vi "setSweepConfiguration.vi"(8 "error in (no error)":errorcluster, 10 "setSweepConfiguration":variant, 11 "Instrument.LockinAPI in":refnum<class "Instrument.LockinAPI.lvclass">) -> (0 "error out":errorcluster, 3 "Instrument.LockinAPI out":refnum<class "Instrument.LockinAPI.lvclass">)   [LabVIEW 2019, in "Instrument.LockinAPI.lvclass"]
doc: "Configure Sweep mode"
uses:
  Instrument.LockinAPI.lvclass
  C:/Users/patrick/Documents/GitHub/Instrument-Framework/lvsrc/Instrument/Instrument.lvclass
  Typedefs/API/LockinAPI.Commands--Enum.ctl
  de6fb303-8df8-49ef-b17e-c3f9f1bf9765.vi
  de6fb303-8df8-49ef-b17e-c3f9f1bf9765.vi/18aa9fab-8d34-42d7-9854-65ef5eaa2568.vi
  de6fb303-8df8-49ef-b17e-c3f9f1bf9765.vi/18aa9fab-8d34-42d7-9854-65ef5eaa2568.vi/384e9f5b-745a-4fe9-8395-b24d125153c2.vi
  de6fb303-8df8-49ef-b17e-c3f9f1bf9765.vi/18aa9fab-8d34-42d7-9854-65ef5eaa2568.vi/384e9f5b-745a-4fe9-8395-b24d125153c2.vi/a2febbde-3d5a-455a-bb03-93f8f6d728bf.vi
  de6fb303-8df8-49ef-b17e-c3f9f1bf9765.vi/18aa9fab-8d34-42d7-9854-65ef5eaa2568.vi/384e9f5b-745a-4fe9-8395-b24d125153c2.vi/28684123-1cf5-4cee-a4b2-57f2f2fe93a2.vi
  Instrument/Protected/Validate API method.vi
  Instrument/Private/Get RC Connection Status.vi
  Instrument/API/Send and Receive.vi
  <vilib>/Utility/Data Type/Get Type Information.vi
  <vilib>/JDP Science/JSONtext/JSON text to Variant.vi
  <vilib>/JDP Science/JSONtext/LVClass Serializer/JSONtext LVClass Serializer.lvclass
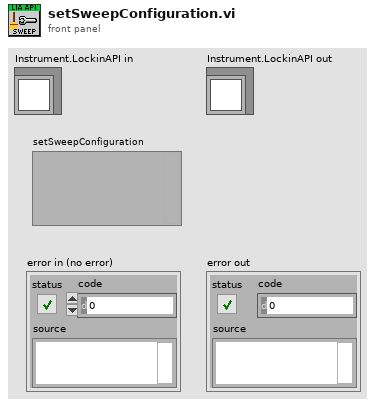
[diagram p1: front panel]
types:
  T1 = typedef "Instrument.LockinAPI.lvclass/LockinAPI.Commands--Enum.ctl" = enum16{"setAI", "setAO", "setAO_Amplitude", "setAO_DC", "setAO_Frequency", "setAO_Phase", "setAO_Function", "setAO_I+", "setREF", "setREF_Frequency", "setREF_Phase", "setREF_TC", "setREF_Roll-Off", "setDAQ", "setSampling", "setOffset", "setState", "getState", "getAO", "getAI", "getResults", "getSampling", "getAOconfig", "getREFconfig", "setInputGain", "setOutputGain", "getInputGain", "getOutputGain", "setSamplingMode", "getSamplingMode", "setSweep", "setSweepTime", "setSweepTable", "getStatus", "getSweepResults", "getSweepWaveforms", "startSweep", "stopSweep", "setAUX", "getAUX"}
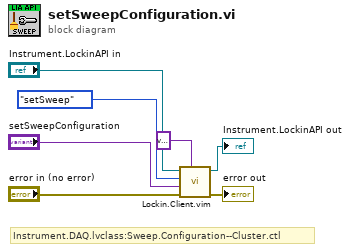
[diagram p0: block diagram]
diagram:
  # "Instrument.DAQ.lvclass:Sweep.Configuration--Cluster.ctl"
  n1 = call "Lockin.Client.vim"("Data Out type"=variant, "error in (no error)"="error in (no error)", "Data"="setSweepConfiguration", "Command"=LockinAPI.Commands--Enum."setSweep", "Instrument.LockinAPI in"="Instrument.LockinAPI in") -> ("error out"=→"error out":errorcluster, "Instrument.LockinAPI out"=→"Instrument.LockinAPI out":refnum<class "Instrument.LockinAPI.lvclass">)  [unwired: 4 in, 1 out]
